vi "Encoder and Gyro Drive Straight.vi"   [LabVIEW 2016]
types:
  T1 = typedef "WPI_GyroDevRef.ctl" = cluster{"DevStatus":errorcluster, "Analog Channel":T2, "Offset":dbl, "Gain (VoltsPerDegree/Second)":dbl, "Gyro Type":enum16{"Analog", "XRS450"}, "Handle":i32, "SPI Bus":T3, "Device Found":bool, "Sample Rate":dbl, "Calibrate On Open":bool}
  T2 = typedef "FPGA_AIChannel.ctl" = enum8{"AI 0", "AI 1", "AI 2", "AI 3", "AI MXP 0", "AI MXP 1", "AI MXP 2", "AI MXP 3", "Invalid"}
  T3 = typedef "spi_bus.ctl" = enum16{"SPI On-Board, CS0", "SPI On-Board, CS1", "SPI On-Board, CS2", "SPI On-Board, CS3", "SPI MXP", "Invalid"}
  T4 = typedef "WPI_MotorControlDeviceRef.ctl" = cluster{"DeviceStatus":errorcluster, "Type":T5, "PWM":cluster{"PWM Channel":T6, "DeadBand":T7}, "CAN":cluster{"Device Number":u8, "SetOutput VI Ref":variant, "GetOutput VI Ref":variant, "Enable VI Ref":variant, "Disable VI Ref":variant, "Data":variant}, "Invert":bool}
  T5 = typedef "WPI_MotorControlType.ctl" = enum16{"PWM", "CAN"}
  T6 = typedef "FPGA_DIOPWMChannel.ctl" = enum8{"PWM 0", "PWM 1", "PWM 2", "PWM 3", "PWM 4", "PWM 5", "PWM 6", "PWM 7", "PWM 8", "PWM 9", "PWM MXP 0", "PWM MXP 1", "PWM MXP 2", "PWM MXP 3", "PWM MXP 4", "PWM MXP 5", "PWM MXP 6", "PWM MXP 7", "PWM MXP 8", "PWM MXP 9", "Invalid"}
  T7 = typedef "WPI_PWMDeadband.ctl" = cluster{"Name":string, "maxPositivePwm":i32, "minPositivePwm":i32, "centerPwm":i32, "maxNegativePwm":i32, "minNegativePwm":i32, "angularRange":u16}
  T8 = typedef "WPI_CANTalonSRX_GlobalStatus.ctl" = cluster{"Applied Throttle":dbl, "Module Enabled":bool, "CAN Error":errorcluster, "Closed Loop Error":dbl, "Forward Limit Switch Closed":bool, "Reverse Limit Switch Closed":bool, "Sensor Position":dbl, "Sensor Velocity":dbl, "Current":dbl, "Sticky Fault - Over Temp":bool, "Sticky Fault - Under Voltage":bool, "Sticky Fault - Forward Limit":bool, "Sticky Fault - Reverse Limit":bool, "Sticky Fault - Forward Soft Limit":bool, "Sticky Fault - Reverse Soft Limit":bool, "Brake is Enabled":bool, "Encoder Position":dbl, "Encoder Velocity":dbl, "Encoder Index Count":dbl, "Encoder A Pin State":bool, "Encoder B Pin State":bool, "Encoder Index Pin State":bool, "Analog In":dbl, "Analog In Velocity":dbl, "Temperature (C)":dbl, "Battery Voltage":dbl, "Control 5 Is Supported":bool, "Current Profile Slot Select":dbl, "Pos Div 8":bool, "Vel Div 4":bool, "Pulse Width Position":i32, "Pulse Width Velocity":i32, "Pulse Width Rise To Rise (us)":i32, "Pulse Width Rise To Fall (us)":i32, "Mot Prof Active Is Under Run":bool, "Mot Prof Active Has Under Run":bool, "Mot Prof Active Is Last":bool, "Mot Prof Active Velocity Only":bool, "Mot Prof Active Is Valid":bool, "Mot Prof Buffer Is Full":bool, "Mot Prof Active Profile Slot Select":i32, "Mot Prof NextID":i32, "Mot Prof Count":i32, "Mot Prof Active Velocity":dbl, "Mot Prof Active Position":dbl, "Mot Prof Output Enable":i32}
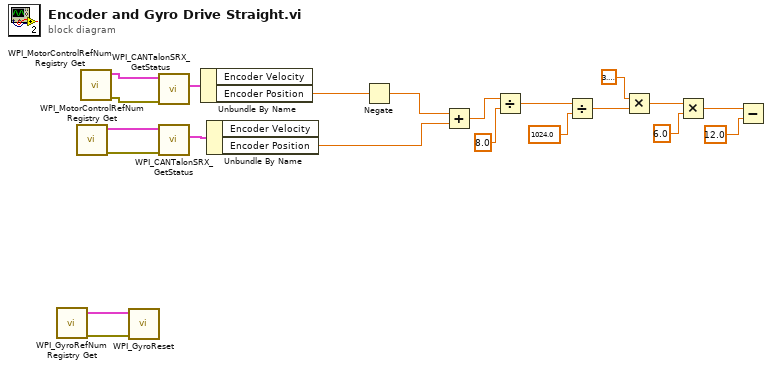
[diagram p0: block diagram]
diagram:
  n1 = call <vilib>:"WPI_GyroRefNum Registry Get.vi"() -> ("error out"=w17:errorcluster, "GyroDevRef"=w18:T1)  [unwired: 10 in]
  n2 = call <vilib>:"WPI_MotorControlRefNum Registry Get.vi"() -> ("error out"=w15:errorcluster, "MotorControlDevRef"=w14:T4)  [unwired: 10 in]
  n3 = call <vilib>:"WPI_MotorControlRefNum Registry Get.vi"() -> ("error out"=w20:errorcluster, "MotorControlDevRef"=w21:T4)  [unwired: 10 in]
  n4 = call <vilib>:"WPI_GyroReset.vi"("error in"=w17, "GyroDevRef"=w18) -> ()  [unwired: 8 in, 2 out]
  n5 = call <vilib>:"WPI_CANTalonSRX_GetStatus.vi"("error in (no error)"=w20, "CAN Talon SRX Ref"=w21) -> ("Talon SRX Status"=w19:T8)  [unwired: 7 in, 2 out]
  n6 = call <vilib>:"WPI_CANTalonSRX_GetStatus.vi"("error in (no error)"=w15, "CAN Talon SRX Ref"=w14) -> ("Talon SRX Status"=w16:T8)  [unwired: 7 in, 2 out]
  n7 = Unbundle By Name(w19) -> ("Encoder Position"=w12:dbl)  [unwired: 1 out]
  n8 = Unbundle By Name(w16) -> ("Encoder Position"=w13:dbl)  [unwired: 1 out]
  n9 = Negate(x=w12) -> (-x=w11:dbl)
  n10 = Add(x=w11, y=w13) -> (x+y=w1:dbl)
  n11 = Divide(x=w1, y=8.0) -> (x/y=w9:dbl)
  n12 = Divide(x=w9, y=1024.0) -> (x/y=w7:dbl)
  n13 = Multiply(x=3.141592653589793, y=w7) -> (x*y=w5:dbl)
  n14 = Multiply(x=w5, y=6.0) -> (x*y=w3:dbl)
  n15 = Subtract(x=w3, y=12.0) -> ()  [unwired: 1 out]
